vi "Main - On Delete.vi"(6 "All deleted Refs":T1[](array[typedef]) format="%.0x", 8 "error in (no error)":errorcluster, 11 "Item Ref in":T1 format="%.0x") -> (0 "error out":errorcluster, 3 "Item Ref out":T1 format="%.0x")   [LabVIEW 2016, in "Scan Engine Custom Device.lvlib"]
uses:
  Scan Engine Custom Device.lvlib
  Type Defs/Host - FPGAScanInterfaceMode.ctl
  <vilib>/NI Veristand/Custom Device Tools/Custom Device Utility Library/Custom Device Utility Library.lvlib
  <vilib>/NI Veristand/Custom Device Tools/Custom Device Utility Library/NI VeriStand - Search for Item by GUID.vi
  Globals/Scan Engine GUIDs.vi
  <vilib>/NI Veristand/Custom Device API/Custom Device Item Ref.ctl
  <vilib>/NI Veristand/Custom Device API/Custom Device API.lvlib
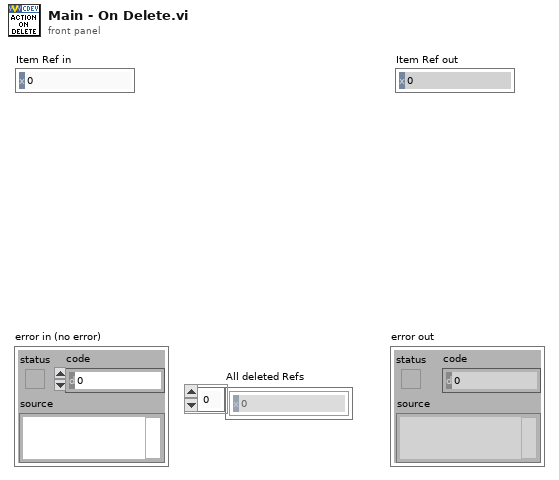
[diagram p1: front panel]
types:
  T1 = typedef "Custom Device API.lvlib/Custom Device Item Ref.ctl" = u64
  T2 = typedef "Scan Engine Custom Device.lvlib/Host - FPGAScanInterfaceMode.ctl" = enum16{"Use Current", "FPGA", "Scan Mode"}
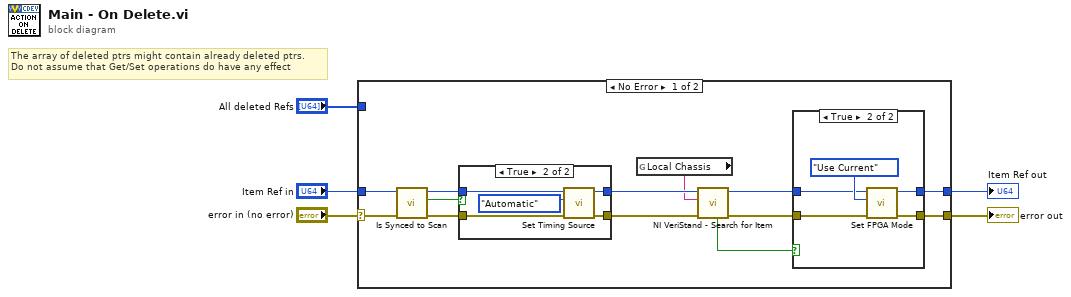
[diagram p0: block diagram]
diagram:
  # "The array of deleted ptrs might contain already deleted ptrs.\nDo not assume that Get/Set operations do have any effect"
  n1 = case shown="No Error" "error in (no error)" {
    selector: "error in (no error)" -> [w17 w34]
    tunnel: [w7 w34] -> w4
    tunnel: "Item Ref in" -> [w18 w33]
    tunnel: [w6 w33] -> w2
    tunnel: "All deleted Refs" -> [_ _]
    frame No Error {
      n2 = call "Is Synced to Scan.vi"("error in"=w17, "Item Ref in"=w18) -> ("error out"=w14:errorcluster, "Sync to Scan?"=w16:bool, "Item Ref out"=w15:T1)  [unwired: 6 in, 1 out]
      n3 = case shown="True" w16 {
        tunnel: w15 -> [w26 w32]
        tunnel: w14 -> [w27 w30]
        tunnel: [w27 w29] -> w12
        tunnel: [w26 w28] -> w13
        frame False {
        }
        frame True {
          n4 = call "Set Timing Source.vi"("error in (no error)"=w30, "Timing Source"=enum16{"Automatic", "Custom Device"}."Automatic", "Item Ref in"=w32) -> ("error out"=w29:errorcluster, "Item Ref out"=w28:T1)  [unwired: 7 in]
        }
      }
      n5 = global read "Scan Engine GUIDs.vi" "Local Chassis"() -> (w11:string)
      n6 = call-poly <vilib>:"NI VeriStand - Search for Item.vi"("error in"=w12, "Item GUID"=w11, "Section Ref in"=w13) -> ("error out"=w8:errorcluster, "Section Ref out"=w9:T1, "Found"=w10:bool)  [unwired: 5 in, 1 out]
      n7 = case shown="True" w10 {
        tunnel: w9 -> [w20 w24]
        tunnel: w8 -> [w19 w23]
        tunnel: [w19 w22] -> w7
        tunnel: [w20 w21] -> w6
        frame False {
        }
        frame True {
          n8 = call "Set FPGA Mode.vi"("error in (no error)"=w23, "FPGAScanInterfaceMode"=Host_-_FPGAScanInterfaceMode."Use Current", "Item Ref in"=w24) -> ("error out"=w22:errorcluster, "Item Ref out"=w21:T1)  [unwired: 7 in]
        }
      }
    }
    frame Error {
    }
  }
  "error out" <- w4
  "Item Ref out" <- w2
